vi "FilterWiresByConnectedTerminals.vi"(7 "Filter wires? (t)":bool=TRUE, 8 "error in (no error)":errorcluster, 10 "Excluded objects":refnum<vi>[](array[refnum]), 11 "Wires in":refnum<vi>[](array[refnum])) -> (0 "error out":errorcluster, 3 "Wires out (filtered)":refnum<vi>[](array[refnum]))   [LabVIEW 2017, in "ErrorStructureDrawer.lvlib"]
doc: "Filter the array of wires: remove any wire from the array if it is connected to any object(s) in the exluded array.\n\nAlso casts the wire references to a more generic type (GObject), even if the filtering is disabled (all input elements are returned in that case)."
uses:
  ErrorStructureDrawer.lvlib
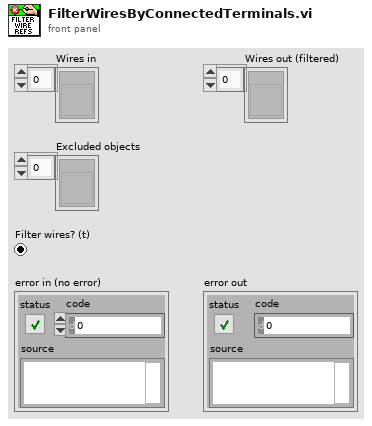
[diagram p1: front panel]
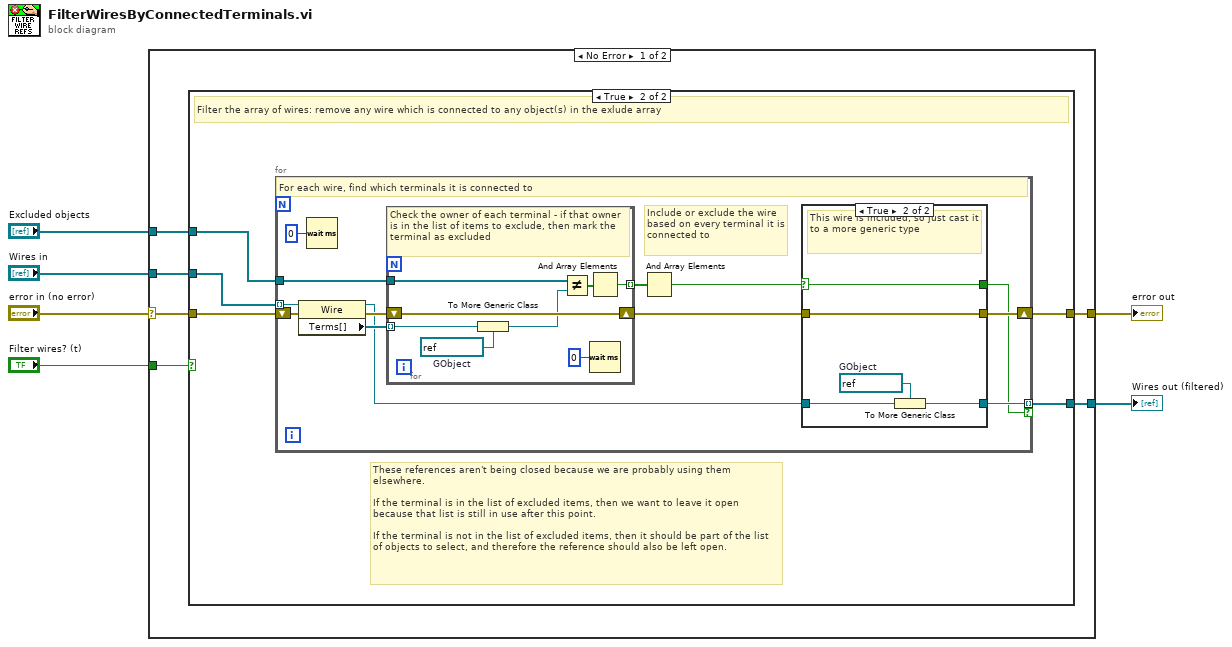
[diagram p0: block diagram]
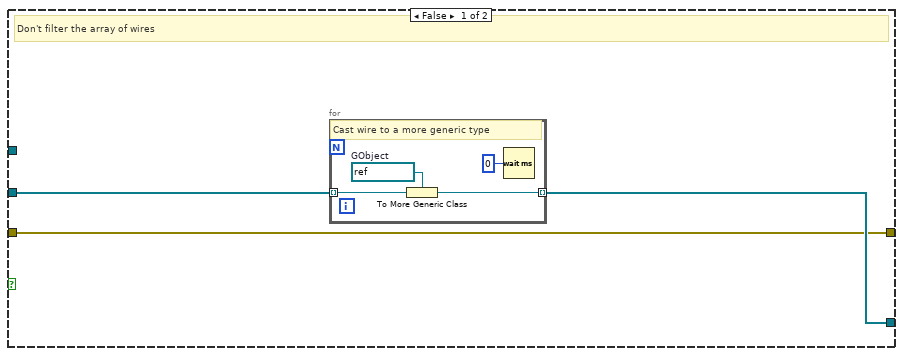
[diagram p2: hidden frame]
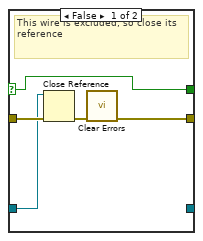
[diagram p3: hidden frame]
diagram:
  n1 = case shown="No Error" "error in (no error)" {
    selector: "error in (no error)" -> [w7 w56]
    tunnel: [w12 _] -> w6
    tunnel: "Filter wires? (t)" -> [w11 _]
    tunnel: [w10 w56] -> w4
    tunnel: "Excluded objects" -> [w9 _]
    tunnel: "Wires in" -> [w8 _]
    frame No Error {
      n2 = case shown="True" w11 {
        tunnel: w8 -> [w15 w24]
        tunnel: w9 -> [_ w20]
        tunnel: [w14 w23] -> w12
        tunnel: [w13 w22] -> w10
        tunnel: w7 -> [w13 w21]
        frame False {
          # "Don't filter the array of wires"
          n3 = for {
            tunnel: w15 -> [w18] mode=indexing
            tunnel: [w17] -> w14 mode=indexing
            w19 = refnum<vi> refnum  # GObject
            # "Cast wire to a more generic type"
            n4 = To More Generic Class(target class=w19, reference=w18) -> (generic class reference=w17:refnum<vi>)
            n5 = Wait (ms)(milliseconds to wait=u32 0) -> ()  [unwired: 1 out]
          }
        }
        frame True {
          # "These references aren't being closed because we are probably using them elsewhere.\n\nIf the terminal is in the list of excluded items, then we want to leave it open because that list is still in use after this point.\n\nIf the terminal is not in the list of excluded items, then it should be part of the list of objects to select, and therefore the reference should also be left open."
          # "Filter the array of wires: remove any wire which is connected to any object(s) in the exlude array"
          n6 = for {
            tunnel: w24 -> [w36] mode=indexing
            tunnel: w20 -> [w34]
            shift-right: [w28] -> w22
            shift-left: w21 -> [w33]
            tunnel: [w27] -> w23 mode=indexing if=w26
            # "Include or exclude the wire based on every terminal it is connected to"
            # "For each wire, find which terminals it is connected to"
            n7 = property class="Wire"(reference=w36, error in=w33) -> (reference out=w29:refnum<vi>, error out=w35:errorcluster, "Terms[]"=w37:refnum<vi>[])
            n8 = Wait (ms)(milliseconds to wait=u32 0) -> ()  [unwired: 1 out]
            n9 = for {
              tunnel: w37 -> [w50] mode=indexing
              tunnel: w34 -> [w54]
              shift-right: [w52] -> w31
              shift-left: w35 -> [w52]
              tunnel: [w53] -> w32 mode=indexing
              w51 = refnum<vi> refnum  # GObject
              # "Check the owner of each terminal - if that owner is in the list of items to exclude, then mark the terminal as excluded"
              n10 = To More Generic Class(target class=w51, reference=w50) -> (generic class reference=w49:refnum<vi>)
              n11 = Not Equal?(x=w54, y=w49) -> (x != y?=w55:bool[])
              n12 = And Array Elements(Boolean array=w55) -> (logical AND=w53:bool)
              n13 = Wait (ms)(milliseconds to wait=u32 0) -> ()  [unwired: 1 out]
            }
            n14 = And Array Elements(Boolean array=w32) -> (logical AND=w30:bool)
            n15 = case shown="True" w30 {
              selector: w30 -> [w38 w44]
              tunnel: w31 -> [w42 w45]
              tunnel: w29 -> [w41 w46]
              tunnel: [w39 w45] -> w28
              tunnel: [w38 w44] -> w26
              tunnel: [_ w43] -> w27
              frame False {
                # "This wire is excluded, so close its reference"
                n16 = Close Reference(reference=w41, error in (no error)=w42) -> (error out=w40:errorcluster)
                n17 = call <vilib>:"Clear Errors.vi"("error in (no error)"=w40) -> ("error out"=w39:errorcluster)  [unwired: 5 in, 1 out]
              }
              frame True {
                w47 = refnum<vi> refnum  # GObject
                # "This wire is included, so just cast it to a more generic type"
                n18 = To More Generic Class(target class=w47, reference=w46) -> (generic class reference=w43:refnum<vi>)
              }
            }
          }
        }
      }
    }
    frame Error {
    }
  }
  "error out" <- w4
  "Wires out (filtered)" <- w6
